vi "Read Hardware Handles.vi"(8 "error in":errorcluster, 11 "AIM ARINC-429 execution unit in":refnum<class "Execution Unit.lvclass">) -> (0 "error out":errorcluster, 2 "hardware handles":T1, 3 "AIM ARINC-429 execution unit out":refnum<class "Execution Unit.lvclass">)   [LabVIEW 2020, in "AIM ARINC 429 Engine.lvlib" / "Implementation.lvlib" / "Execution Unit.lvclass"]
uses:
  Execution Unit.lvclass
  Custom Device/Hardware Handles.ctl
  Custom Device/Custom Device.lvlib
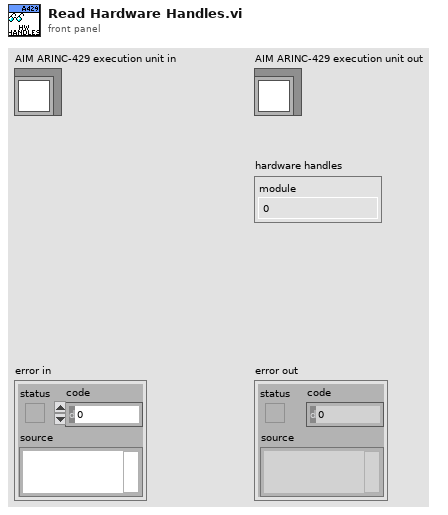
[diagram p1: front panel]
types:
  T1 = typedef "AIM ARINC 429 Engine.lvlib/Custom Device.lvlib/Hardware Handles.ctl" = cluster{"module":u8}
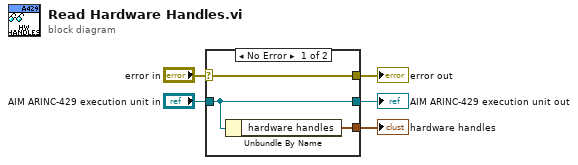
[diagram p0: block diagram]
diagram:
  n1 = case shown="No Error" "error in" {
    selector: "error in" -> [w8 w9]
    tunnel: [w8 w9] -> w4
    tunnel: [w7 w10] -> w2
    tunnel: "AIM ARINC-429 execution unit in" -> [w7 w10]
    tunnel: [w6 _] -> w1
    frame No Error {
      n2 = Unbundle By Name(w7) -> ("hardware handles"=w6:T1)
    }
    frame Error {
    }
  }
  "error out" <- w4
  "AIM ARINC-429 execution unit out" <- w2
  "hardware handles" <- w1
